vi "Write Send Binary Data.vi"(8 "error in (no error)":errorcluster, 9 "values":u8[](array[numeric]), 10 "starting address":u16, 11 "standard data model in":refnum<class "WebSocket Data Model.lvclass">) -> (0 "error out":errorcluster, 3 "standard data model out":refnum<class "WebSocket Data Model.lvclass">)   [LabVIEW 2021, in "WebSockets.lvlib" / "WebSocket Data Model.lvclass"]
doc: "Writes the values of multiple input register values in series, starting at address M."
uses:
  WebSocket Data Model.lvclass
  WebSocket Data Model.lvclass/WebSocket Data Model.ctl
  WebSocket/Opcodes.ctl
  WebSocket/WebSocket.lvclass
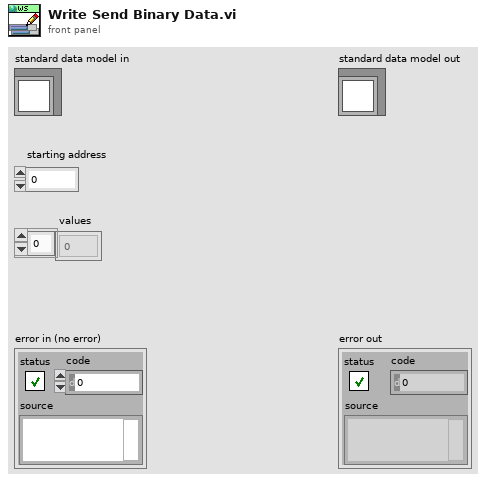
[diagram p1: front panel]
types:
  T1 = typedef "WebSockets.lvlib/WebSocket.lvclass/Opcodes.ctl" = u8
  T2 = typedef "WebSockets.lvlib/WebSocket Data Model.lvclass/Data Model.ctl" = cluster{"UTC":u64, "Receive Binary Data":u8[], "Receive Text Data":string, "Send Binary Data":u8[], "Send Text Data":string, "ES":u8}
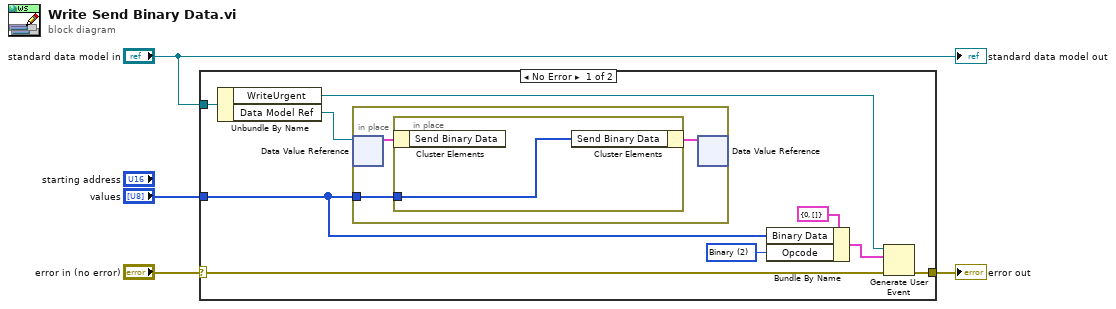
[diagram p0: block diagram]
diagram:
  n1 = case shown="No Error" "error in (no error)" {
    selector: "error in (no error)" -> [w10 w18]
    tunnel: "values" -> [w6 _]
    tunnel: "standard data model in" -> [w13 _]
    tunnel: [w9 w18] -> w2
    frame No Error {
      w7 = T1 2 items=["Cont. Frame"=0, "Text"=1, "Binary"=2, "Close Frame"=8, "Ping"=9, "Pong"=10] ("Opcode")
      n2 = Unbundle By Name(w13) -> ("WriteUrgent"=w11:refnum<user-event>, "Data Model Ref"=w12:refnum<data-value>)
      n3 = in-place {
        in-place-border: w6 -> [w16]
        n4 = in-place-dvr #1(w12) -> (w15:T2)  [unwired: 1 out]
        n5 = in-place {
          in-place-border: w16 -> [w17]
          n6 = in-place-cluster #2(w15) -> ()  [unwired: 1 out]
          n7 = in-place-cluster #2("Send Binary Data"=w17) -> (w14:T2)
        }
        n8 = in-place-dvr #1(w14) -> ()  [unwired: 2 out]
      }
      n9 = Bundle By Name(cluster=cluster{"Opcode":T1, "Binary Data":u8[]} {"Opcode"=0, "Binary Data"=[]} ("Data"), "Binary Data"=w6, "Opcode"=w7) -> (w5:cluster{"Opcode":T1, "Binary Data":u8[]})
      n10 = Generate User Event(user event=w11, event data cluster=w5, error in=w10) -> (error out=w9:errorcluster)  [unwired: 1 in, 1 out]
    }
    frame Error {
    }
  }
  "error out" <- w2
  "standard data model out" <- "standard data model in"
